vi "AB_Source_Delete_Save_Settings.vi"(8 "error in (no error)":errorcluster, 11 "sourceProperties in":T1[](array[typedef])) -> (0 "error out":errorcluster, 1 "saveSettings":T1[](array[typedef]), 2 "found":bool, 3 "sourceProperties out":T1[](array[typedef]))   [LabVIEW 2020]
uses:
  <vilib>/AppBuilder/AB_Source_Properties.ctl
  <vilib>/AppBuilder/AB_Source_Property_Type.ctl
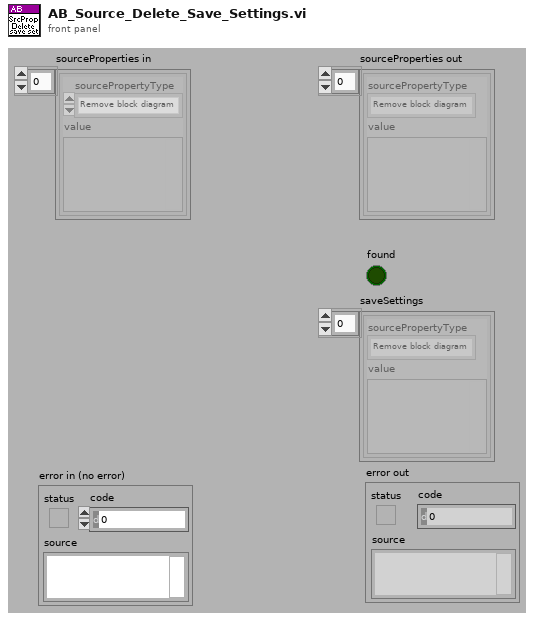
[diagram p1: front panel]
types:
  T1 = typedef "AB_Source_Properties.ctl" = cluster{"sourcePropertyType":T2, "value":variant}
  T2 = typedef "AB_Source_Property_Type.ctl" = enum16{"Remove block diagram", "Remove front panel", "Password", "Window has title bar", "Show menu bar", "Show vertical scroll bar", "Show horizontal scroll bar", "Show toolbar", "Show Abort button", "Show fp when called", "Window behavior", "Allow user to close window", "Window run-time position", "Run when opened", "Allow debugging", "Auto error handling", "Generate guard code", "Use stack variables", "Expression folding", "Integer only", "Inline subVI"}
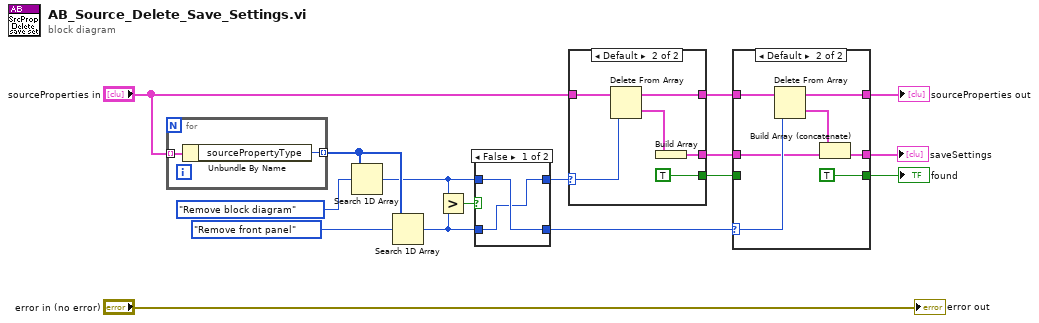
[diagram p0: block diagram]
diagram:
  n1 = for {
    tunnel: "sourceProperties in" -> [w18] mode=indexing
    tunnel: [w17] -> w14 mode=indexing
    n2 = Unbundle By Name(w18) -> ("sourcePropertyType"=w17:T2)
  }
  n3 = Search 1D Array(1D array=w14, element=AB_Source_Property_Type."Remove block diagram") -> (index of element=w10:i32)  [unwired: 1 in]
  n4 = Search 1D Array(1D array=w14, element=AB_Source_Property_Type."Remove front panel") -> (index of element=w9:i32)  [unwired: 1 in]
  n5 = Greater?(x=w10, y=w9) -> (0:w11:bool)
  n6 = case shown="False" w11 {
    tunnel: [w19 w22] -> w8
    tunnel: w10 -> [w20 w22]
    tunnel: [w20 w21] -> w5
    tunnel: w9 -> [w19 w21]
    frame False {
    }
    frame True {
    }
  }
  n7 = case shown="Default" w8 {
    selector: w8 -> [_ w26]
    tunnel: "sourceProperties in" -> [w23 w28]
    tunnel: [_ TRUE] -> w1
    tunnel: [w23 w27] -> w7
    tunnel: [_ w24] -> w4
    frame -1 {
    }
    frame Default {
      n8 = Delete From Array(array=w28, index=w26) -> (deleted portion=w25:T1, array with subset deleted=w27:T1[])  [unwired: 1 in]
      n9 = Build Array(w25) -> (w24:T1[])
    }
  }
  n10 = case shown="Default" w5 {
    selector: w5 -> [_ w36]
    tunnel: w7 -> [w32 w38]
    tunnel: [w30 TRUE] -> w3
    tunnel: [w32 w37] -> w6
    tunnel: [w31 w34] -> w2
    tunnel: w4 -> [w31 w33]
    tunnel: w1 -> [w30 _]
    frame -1 {
    }
    frame Default {
      n11 = Delete From Array(array=w38, index=w36) -> (deleted portion=w35:T1, array with subset deleted=w37:T1[])  [unwired: 1 in]
      n12 = Build Array (concatenate)(w35, w33) -> (w34:T1[])
    }
  }
  "sourceProperties out" <- w6
  "found" <- w3
  "saveSettings" <- w2
  "error out" <- "error in (no error)"
